vi "MutationParentLevelsRemoved.vi"(8 "error in (no error)":errorcluster, 10 "Parent Levels Removed":u16, 11 "SerializedClassHeader (child,parent)":T5[](array[typedef])) -> (0 "error out":errorcluster, 2 "ClassOps":T1[](array[typedef]), 3 "SerializedClassHeader (child,parent)":T5[](array[typedef]))   [LabVIEW 2019, in "BlueSerialization.lvlib" / "BlueSerializer.lvclass"]
uses:
  BlueSerializer.lvclass
  ClassHeader.ctl
  <vilib>/Utility/EditLVLibs/LibVersion.ctl
  Support/SetSerializableDataClusterIterable.ctl
  BlueSerializable/BlueSerializable.lvclass
  Support/SetSerializableDataClusterLayer.ctl
  BlueSerializableVersion.ctl
  Support/SetSerializableDataObject.ctl
  <vilib>/Utility/EditLVLibs/Edit LVLibs.lvlib
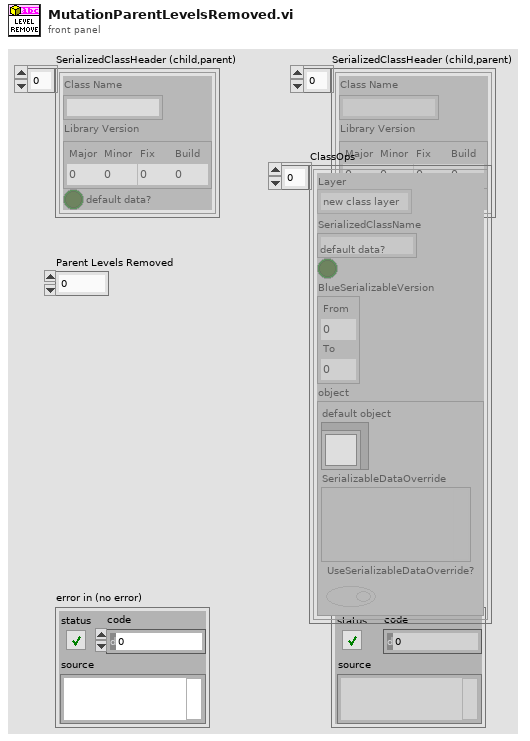
[diagram p1: front panel]
types:
  T1 = typedef "BlueSerialization.lvlib/BlueSerializer.lvclass/SetSerializableDataClusterIterable.ctl" = cluster{"Layer":T2, "SerializedClassName":string, "default data?":bool, "BlueSerializableVersion":T3, "object":T4}
  T2 = typedef "BlueSerialization.lvlib/BlueSerializer.lvclass/SetSerializableDataClusterLayer.ctl" = enum16{"new class layer", "dropped class layer", "agreed class layer"}
  T3 = typedef "BlueSerialization.lvlib/BlueSerializer.lvclass/BlueSerializableVersion.ctl" = cluster{"From":u16, "To":u16}
  T4 = typedef "BlueSerialization.lvlib/BlueSerializer.lvclass/SetSerializableDataObject.ctl" = cluster{"default object":refnum<class "BlueSerializable.lvclass">, "SerializableDataOverride":variant, "UseSerializableDataOverride?":bool}
  T5 = typedef "BlueSerialization.lvlib/BlueSerializer.lvclass/ClassHeader.ctl" = cluster{"Class Name":string, "Library Version":T6, "default data?":bool}
  T6 = typedef "Edit LVLibs.lvlib/LibVersion.ctl" = cluster{"Major":u16, "Minor":u16, "Fix":u16, "Build":u16}
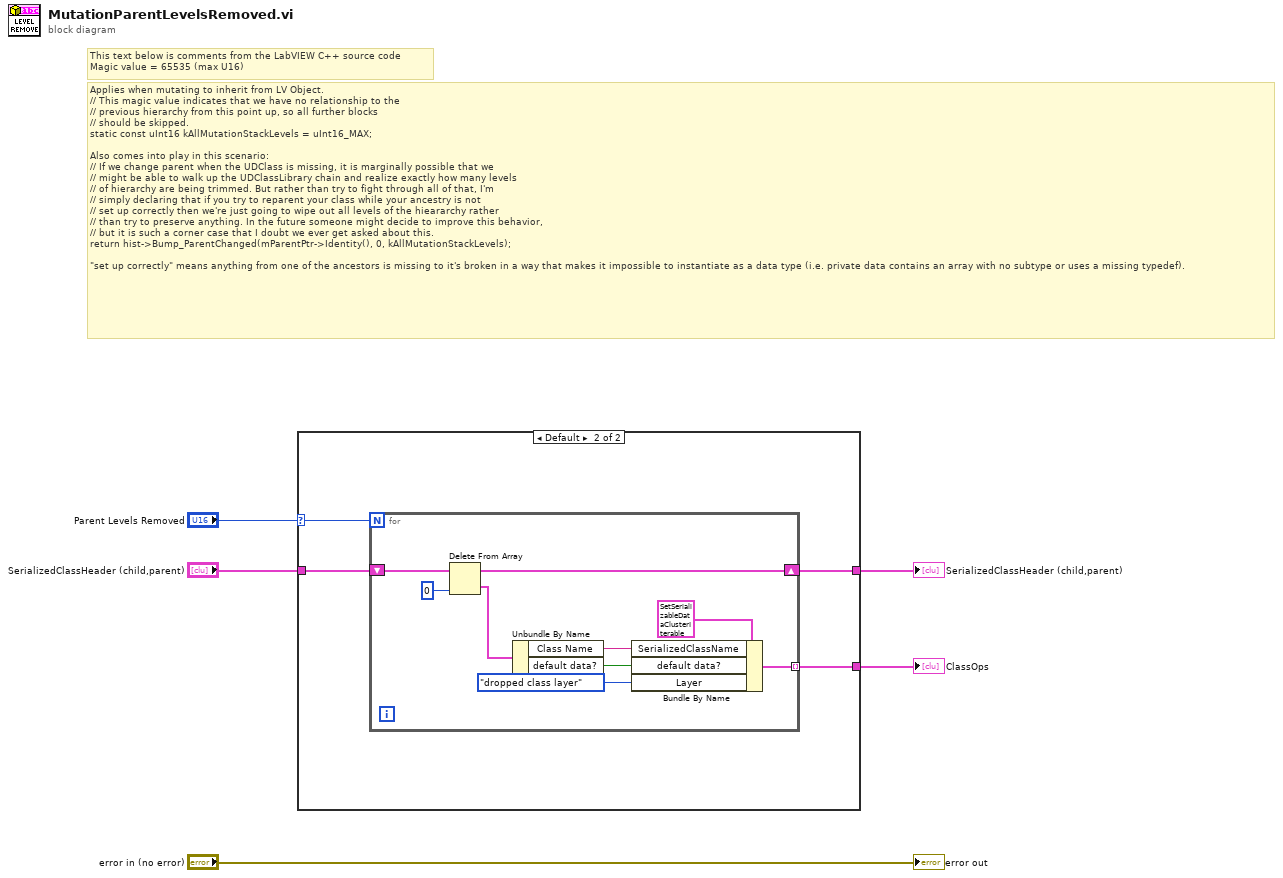
[diagram p0: block diagram]
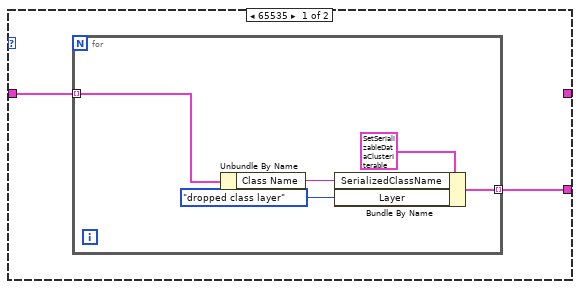
[diagram p2: hidden frame]
diagram:
  # "This text below is comments from the LabVIEW C++ source code\nMagic value = 65535 (max U16)"
  # "Applies when mutating to inherit from LV Object.\n// This magic value indicates that we have no relationship to the\n// previous hierarchy from this point up, so all further blocks\n// should be skipped.\nstatic const uInt16 kAllMutationStackLevels = uInt16_MAX;\n\nAlso comes into play in this scenario:\n// If we change parent when the UDClass is missing, it is marginally possible that we\n// might be able to walk up the UDClassLibrary chain and realize exactly how many levels\n// of hierarchy are being trimmed. But rather than try to fight through all of that, I'm\n// simply declaring that if you try to reparent your class while your ancestry is not\n// set up correctly then we're just going to wipe out all levels of the hieararchy rather\n// than try to preserve anything. In the future someone might decide to improve this behavior,\n// but it is such a corner case that I doubt we ever get asked about this.\nreturn hist->Bump_ParentChanged(mParentPtr->Identity(), 0, kAllMutationStackLevels);\n\n\"set up correctly\" means anything from one of the ancestors is missing to it's broken in a way that makes it impossible to instantiate as a data type (i.e. private data contains an array with no subtype or uses a missing typedef)."
  n1 = case shown="Default" "Parent Levels Removed" {
    selector: "Parent Levels Removed" -> [_ w16]
    tunnel: "SerializedClassHeader (child,parent)" -> [w7 w15]
    tunnel: [_ w14] -> w2
    tunnel: [w6 w13] -> w1
    frame 65535 {
      n2 = for {
        tunnel: [w11] -> w6 mode=indexing
        tunnel: w7 -> [w8] mode=indexing
        n3 = Unbundle By Name(w8) -> ("Class Name"=w9:string)
        n4 = Bundle By Name(cluster=T1 {"Layer"=enum."new class layer", "SerializedClassName"="", "default data?"=FALSE, "BlueSerializableVersion"={"From"=0, "To"=0}, "object"={"default object"=refnum, "SerializableDataOverride"=variant(cluster{"SerializableData":variant, "Use?":bool} {"SerializableData"=variant, "Use?"=FALSE}), "UseSerializableDataOverride?"=FALSE}} ("Cluster 2"), "SerializedClassName"=w9, "Layer"=SetSerializableDataClusterLayer."dropped class layer") -> (w11:T1)
      }
    }
    frame Default {
      n5 = for {
        N: w16 -> [_]
        shift-right: [w23] -> w14
        shift-left: w15 -> [w24]
        tunnel: [w21] -> w13 mode=indexing
        n6 = Delete From Array(array=w24, index=0) -> (deleted portion=w19:T5, array with subset deleted=w23:T5[])  [unwired: 1 in]
        n7 = Unbundle By Name(w19) -> ("Class Name"=w18:string, "default data?"=w17:bool)
        n8 = Bundle By Name(cluster=T1 {"Layer"=enum."new class layer", "SerializedClassName"="", "default data?"=FALSE, "BlueSerializableVersion"={"From"=0, "To"=0}, "object"={"default object"=refnum, "SerializableDataOverride"=variant(cluster{"SerializableData":variant, "Use?":bool} {"SerializableData"=variant, "Use?"=FALSE}), "UseSerializableDataOverride?"=FALSE}} ("Cluster 2"), "SerializedClassName"=w18, "default data?"=w17, "Layer"=SetSerializableDataClusterLayer."dropped class layer") -> (w21:T1)
      }
    }
  }
  "SerializedClassHeader (child,parent)" <- w2
  "ClassOps" <- w1
  "error out" <- "error in (no error)"
